vi "Check if Error Occurred.vi"(8 "error in (no error)":errorcluster, 11 "Response header":string) -> (0 "error out":errorcluster, 3 "Error Occurred":bool)   [LabVIEW 2015, in "NI_Azure_Core.lvlib"]
doc: "Check the response header to see if there was an error.\nIf an error is found, the AWS_S3_Get_Call_Result.vi may get the details from the response body."
uses:
  NI_Azure_Core.lvlib
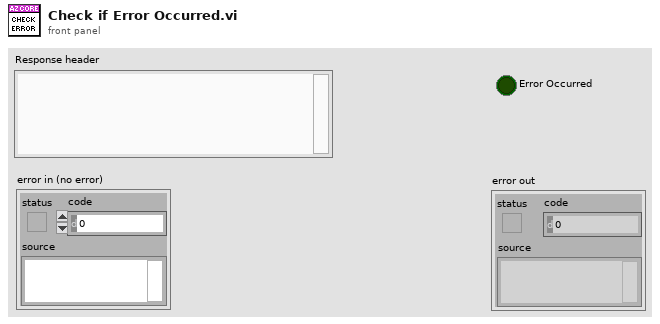
[diagram p1: front panel]
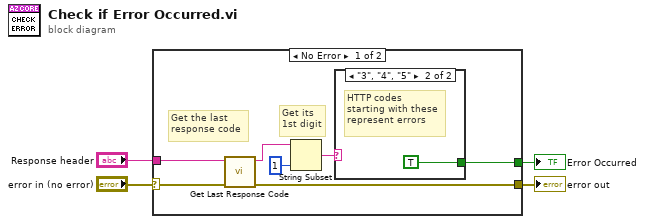
[diagram p0: block diagram]
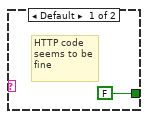
[diagram p2: hidden frame]
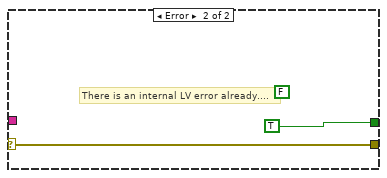
[diagram p3: hidden frame]
diagram:
  n1 = case shown="No Error" "error in (no error)" {
    selector: "error in (no error)" -> [w11 w15]
    tunnel: [w10 w15] -> w2
    tunnel: "Response header" -> [w6 _]
    tunnel: [w5 TRUE] -> w1
    frame No Error {
      # "Get its\n1st digit"
      # "Get the last\nresponse code"
      n2 = call "Get Last Response Code.vi"("error in (no error)"=w11, "Response header"=w6) -> ("error out"=w10:errorcluster, "Response code (last)"=w9:string)  [unwired: 8 in]
      n3 = String Subset(string=w9, length (rest)=1 ("length (rest)")) -> (substring=w8:string)  [unwired: 1 in]
      n4 = case shown="\"3\", \"4\", \"5\"" w8 {
        tunnel: [FALSE TRUE] -> w5
        frame Default {
          # "HTTP code\nseems to be\nfine"
        }
        frame "3", "4", "5" {
          # "HTTP codes\nstarting with these\nrepresent errors"
        }
      }
    }
    frame Error {
      (unwired) FALSE
      # "There is an internal LV error already...."
    }
  }
  "Error Occurred" <- w1
  "error out" <- w2
